vi "Error Check.vi"(8 "error in (no error)":errorcluster, 11 "Keithley 622x2182 Driver in":refnum<class "Keithley 622x2182 Driver.lvclass">) -> (0 "error out":errorcluster, 3 "Keithley 622x2182 Driver out":refnum<class "Keithley 622x2182 Driver.lvclass">)   [LabVIEW 2021, in "Keithley 622x2182 Driver.lvclass"]
uses:
  Keithley 622x2182 Driver.lvclass
  C:/GitHub/NHMFL_Core/Libraries/Instruments/VISA Instrument/VISA Instrument.lvclass
  VISA Instrument/VISA Instrument.lvclass/VISA Instrument.ctl
  VISA Instrument/Read VISA resource.vi
  VISA Instrument/Write VISA resource.vi
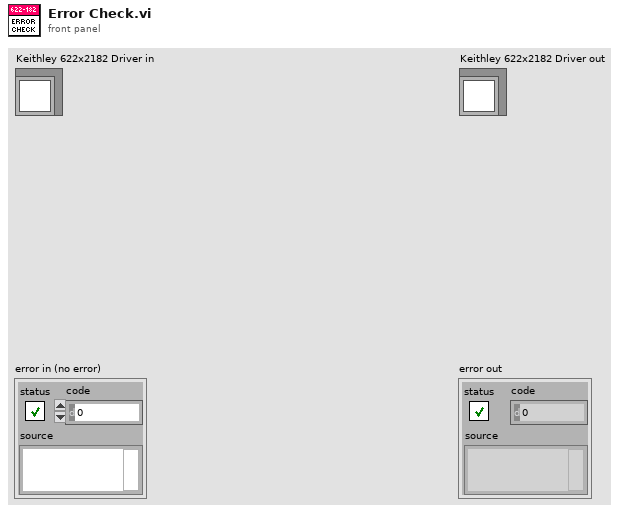
[diagram p1: front panel]
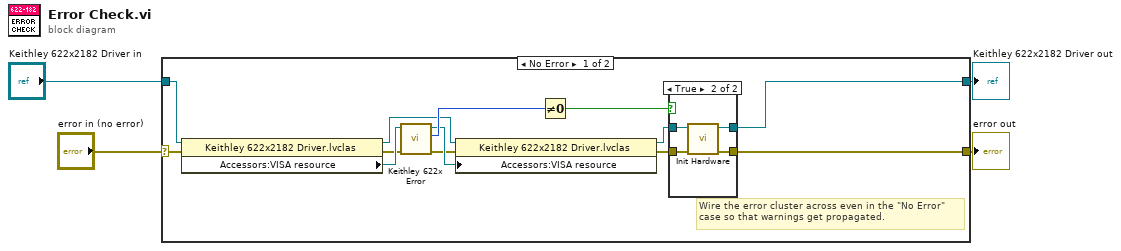
[diagram p0: block diagram]
diagram:
  n1 = case shown="No Error" "error in (no error)" {
    selector: "error in (no error)" -> [w11 w25]
    tunnel: [w10 w25] -> w3
    tunnel: [w6 w24] -> w1
    tunnel: "Keithley 622x2182 Driver in" -> [w5 w24]
    frame No Error {
      # "Wire the error cluster across even in the \"No Error\"\ncase so that warnings get propagated."
      n2 = property class="Keithley 622x2182 Driver.lvclas"(reference=w5, error in=w11) -> (reference out=w14:refnum<class "Keithley 622x2182 Driver.lvclass">, error out=w16:errorcluster, "Accessors:VISA resource"=w17:refnum<visa-resource-name>)
      n3 = call "Keithley 622x Error.vi"("error in"=w16, "VISA resource name"=w17) -> ("error out"=w12:errorcluster, "Error code"=w15:i32, "VISA resource name out"=w13:refnum<visa-resource-name>)  [unwired: 4 in, 3 out]
      n4 = property class="Keithley 622x2182 Driver.lvclas"(reference=w14, error in=w12, "Accessors:VISA resource"=w13) -> (reference out=w9:refnum<class "Keithley 622x2182 Driver.lvclass">, error out=w8:errorcluster)
      n5 = Not Equal To 0?(x=w15) -> (x != 0?=w7:bool)
      n6 = case shown="True" w7 {
        tunnel: [w18 w23] -> w10
        tunnel: w9 -> [w19 w22]
        tunnel: w8 -> [w18 w21]
        tunnel: [w19 w20] -> w6
        frame False {
        }
        frame True {
          n7 = call-dynamic "Init Hardware.vi"("error in (no error)"=w21, "Keithley 622x Driver in"=w22) -> ("error out"=w23:errorcluster, "Keithley 622x Driver out"=w20:refnum<class "Keithley 622x2182 Driver.lvclass">)  [unwired: 8 in]
        }
      }
    }
    frame Error {
    }
  }
  "error out" <- w3
  "Keithley 622x2182 Driver out" <- w1
